vi "plot_data_init.vi"(0 "pixels Y":u32, 1 "pixels X":u32, 3 "active range (%)":u32=98, 5 "error in (no error)":errorcluster) -> (14 "plot data active":i32[][](array[numeric]), 16 "plot data":i32[][](array[numeric]), 17 "Y active idx start":i32, 18 "Y active length":i32, 19 "error out":errorcluster)   [LabVIEW 2010, in "OSA.lvclass"]
doc: "Reads the contents of a <B>Thorlabs_OSA_64</B> object.\n\n[GOOP 1.0]"
uses:
  OSA.lvclass
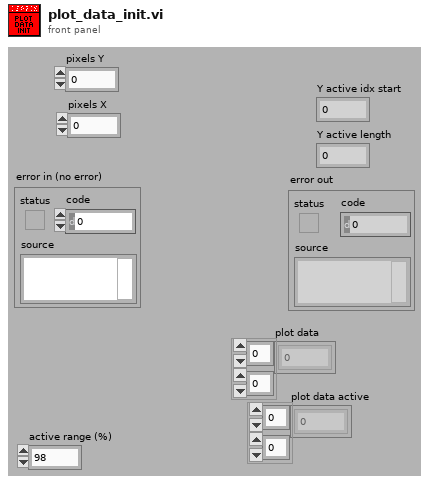
[diagram p1: front panel]
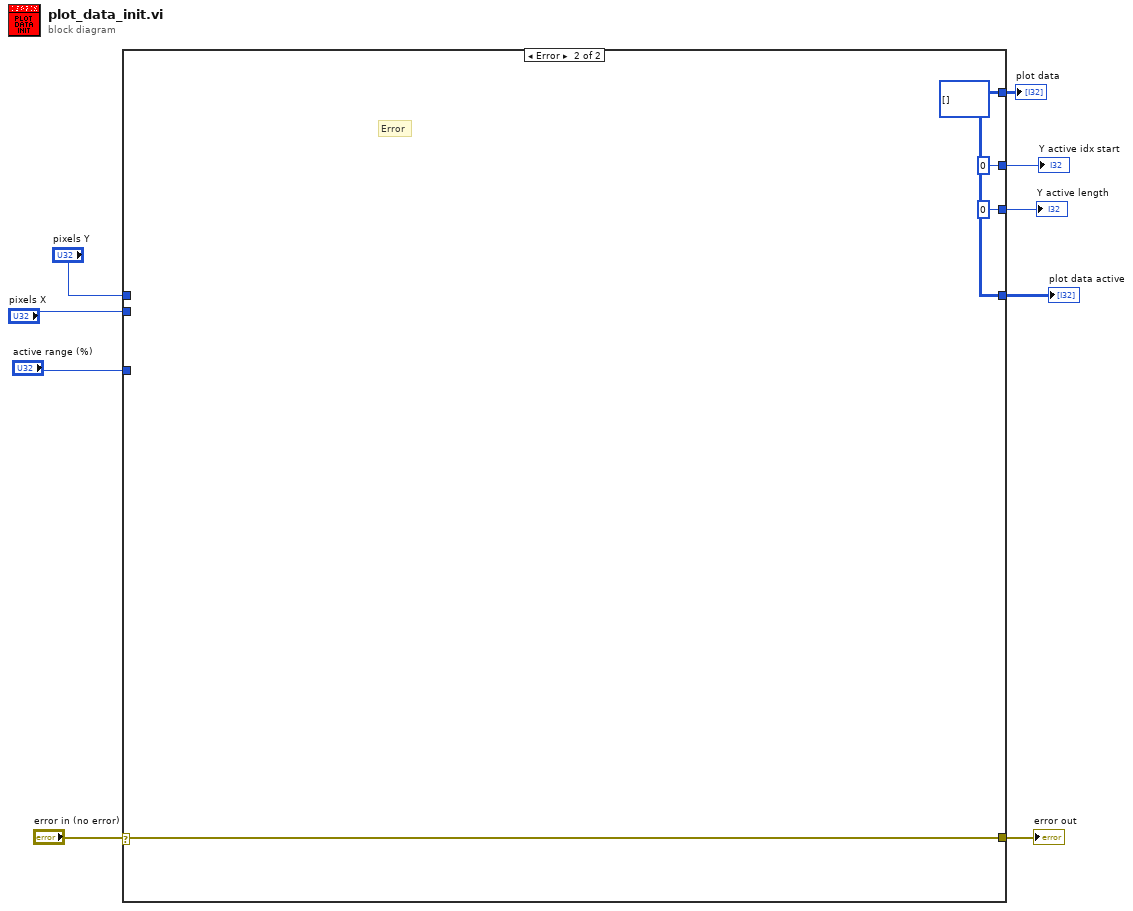
[diagram p0: block diagram]
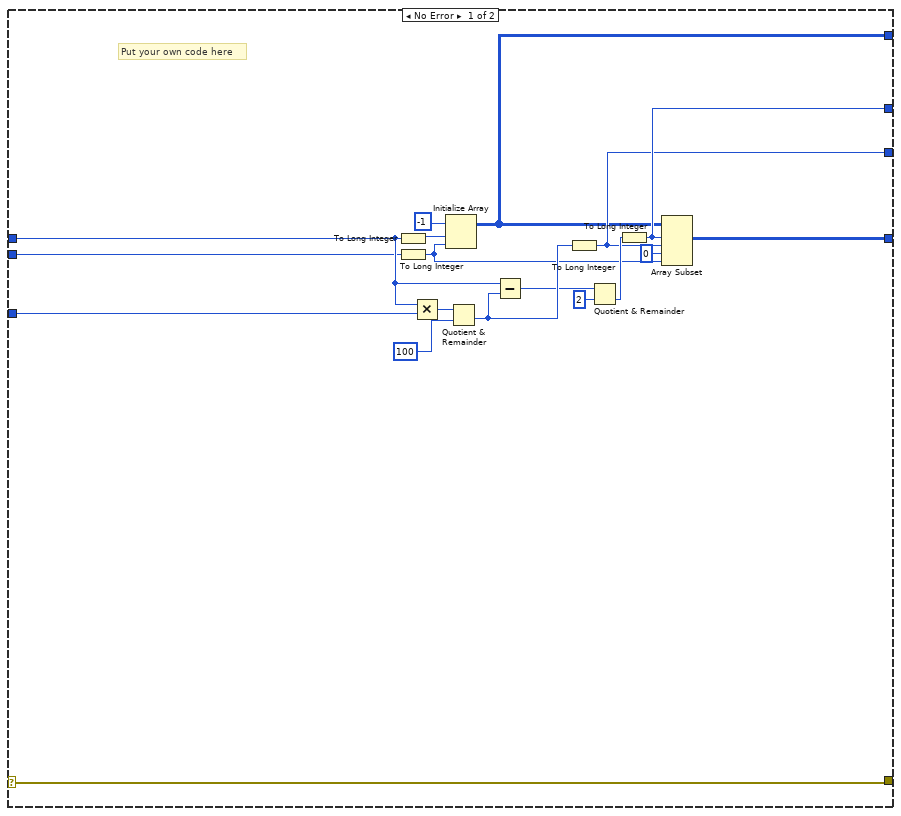
[diagram p2: hidden frame]
diagram:
  n1 = case shown="Error" "error in (no error)" {
    selector: "error in (no error)" -> [w10 w31]
    tunnel: [w10 w31] -> w9
    tunnel: [w16 w30] -> w7
    tunnel: "pixels Y" -> [w21 _]
    tunnel: "pixels X" -> [w20 _]
    tunnel: "active range (%)" -> [w18 _]
    tunnel: [w13 0] -> w3
    tunnel: [w12 0] -> w2
    tunnel: [w11 w30] -> w1
    frame No Error {
      # "Put your own code here"
      n2 = To Long Integer(number=w21) -> (32bit integer=w26:i32)
      n3 = To Long Integer(number=w20) -> (32bit integer=w14:i32)
      n4 = Multiply(x=w21, y=w18) -> (x*y=w25:u32)
      n5 = Initialize Array(-1, w26, w14) -> (w11:i32[][])
      n6 = Quotient & Remainder(x=w25, y=u32 100) -> (floor(x/y)=w24:u32)  [unwired: 1 out]
      n7 = Subtract(x=w21, y=w24) -> (x-y=w23:u32)
      n8 = To Long Integer(number=w24) -> (32bit integer=w12:i32)
      n9 = Quotient & Remainder(x=w23, y=u32 2) -> (floor(x/y)=w22:u32)  [unwired: 1 out]
      n10 = To Long Integer(number=w22) -> (32bit integer=w13:i32)
      n11 = Array Subset(array=w11, index (row)=w13, length (row)=w12, index (col)=0 ("index"), length (col)=w14) -> (w16:i32[][])
    }
    frame Error {
      w30 = i32[][] []
      # "Error"
    }
  }
  "error out" <- w9
  "plot data active" <- w7
  "Y active idx start" <- w3
  "Y active length" <- w2
  "plot data" <- w1
